vi "AmicTimeToShift.vi"(10 "input string":string) -> (2 "s? t:f":string)   [LabVIEW 2012]
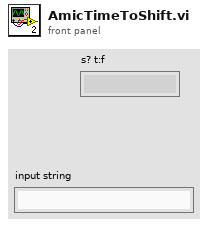
[diagram p1: front panel]
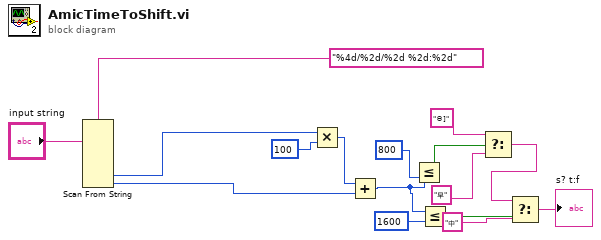
[diagram p0: block diagram]
diagram:
  n1 = Scan From String(format string="%4d/%2d/%2d %2d:%2d", input string="input string") -> (output 4=w2:i32, output 5=w1:i32)  [unwired: 10 in, 3 out]
  n2 = Multiply(x=w2, y=100) -> (x*y=w14:i32)
  n3 = Add(x=w14, y=w1) -> (x+y=w4:i32)
  n4 = Less Or Equal?(x=w4, y=800) -> (x <= y?=w12:bool)
  n5 = Less Or Equal?(x=w4, y=1600) -> (x <= y?=w8:bool)
  n6 = Select(t="©]", s=w12, f="早") -> (s? t:f=w3:string)
  n7 = Select(t=w3, s=w8, f="中") -> (s? t:f=→"s? t:f":string)
